vi "rsidr_core_global.vi"() -> ()   [LabVIEW 2020, in "Rohde&Schwarz CMWXP NR FR1 Measurement.lvlib"] (continued)
position\n\n<10_MErrPeakHighLimCheck>\n limit check result\nMagnitude error peak value, high EVM window position\n\n<11_PErr_RMSlowLimCheck>\n limit check result\nPhase error RMS value, low EVM window position\n\n<12_PErr_RMShLimCheck>\n limit check result\nPhase error RMS value, high EVM window position\n\n<13_PErrPeakLowLimCheck>\n limit check result\nPhase error peak value, low EVM window position\n\n<14_PErrPeakHighLimCheck>\n limit check result\nPhase error peak value, high EVM window position\n\n<15_IQoffsetLimCheck>\n limit check result\nI/Q origin offset\n\n<16_FreqErrorLimCheck>\n limit check result\nCarrier frequency error\n\n<17_TimingErrorLimCheck>\n limit check result\nTransmit time error\n\n<18_TXpowerLimCheck>\n limit check result\nUser equipment power\n\n<19_PeakPowerLimCheck>\n limit check result\nUser equipment peak power\n\n<20_RBpowerLimCheck>\n limit check result\nRB power\n\n<21_EVM_DMRSlLimCheck>\n limit check result\nEVM DMRS value, low EVM window position\n\n<22_EVM_DMRShLimCheck>\n limit check result\nEVM DMRS value, high EVM window position\n\n<23_MErr_DMRSlLimCheck>\n limit check result\nMagnitude error DMRS value, low EVM window position\n\n<24_MErr_DMRShLimCheck>\n limit check result\nMagnitude error DMRS value, high EVM window position\n\n<25_PErr_DMRSLimCheck>\n limit check result\nPhase error DMRS value, low EVM window position\n\n<26_PErr_DMRShLimCheck>\n limit check result\nPhase error DMRS value, high EVM window position\n\n<27_FreqErrorPpmLimCheck>\n limit check result\nCarrier frequency error in ppm\n\n<28_SampleClockELimCheck>\n limit check result\nSample clock error\n\nAvailable Repeated Capabilities:\ninstance: i0, i1, i2, i3, i4, i5, i6, i7, i8, i9, i10, i11, i12, i13, i14, i15, i16, i17, i18, i19, i20, i21, i22, i23, i24, i25, i26, i27, i28, i29, i30, i31, i32\r\n\nRemote-control command(s):\nCALCulate:NRSub:MEAS<i>:MEValuation:MODulation:CURRent?"}, {"Level"=4, "Class Only"=FALSE, "Identifier"="RSCMWXPNRFR1M_ATTR_QUERY_MULTI_EVAL_MEAS_MODULATION_AVERAGE_LIMIT_CHECK_RESULTS", "Descriptive Name"="Query Multi Eval Meas Modulation Average Limit Check Results", "Data Type"=enum."RawString", "Command"="CALC:NRS:MEAS{instance}:MEV:MOD:AVER?", "Access"=enum."Read Only", "Range Table"="", "Read Callback"="", "Write Callback"="", "Range Callback"="", "Check Callback"="", "Rngtable Callback"="", "Coerce Callback"="", "Supported Models"="", "Instrument Options"="", "Check Status Callback"="", "Flags"=0, "Help"="Return the average single value limit check results.\n\nReturn values:  \n<1_Reliability>\n decimal\n\n<2_OutOfTol>\n decimal\nOut of tolerance result, i.e. percentage of measurement intervals of the statistic count for modulation measurements exceeding the specified modulation limits.\n\n<3_EVM_RMSlowLimCheck>\n limit check result\nEVM RMS value, low EVM window position\n\n<4_EVM_RMShighLimCheck>\n limit check result\nEVM RMS value, high EVM window position\n\n<5_EVMpeakLowLimCheck>\n limit check result\nEVM peak value, low EVM window position\n\n<6_EVMpeakHighLimCheck>\n limit check result\nEVM peak value, high EVM window position\n\n<7_MErr_RMSlowLimCheck>\n limit check result\nMagnitude error RMS value, low EVM window position\n\n<8_MErr_RMShighLimCheck>\n limit check result\nMagnitude error RMS value, high EVM window position\n\n<9_MErrPeakLowLimCheck>\n limit check result\nMagnitude error peak value, low EVM window position\n\n<10_MErrPeakHighLimCheck>\n limit check result\nMagnitude error peak value, high EVM window position\n\n<11_PErr_RMSlowLimCheck>\n limit check result\nPhase error RMS value, low EVM window position\n\n<12_PErr_RMShLimCheck>\n limit check result\nPhase error RMS value, high EVM window position\n\n<13_PErrPeakLowLimCheck>\n limit check result\nPhase error peak value, low EVM window position\n\n<14_PErrPeakHighLimCheck>\n limit check result\nPhase error peak value, high EVM window position\n\n<15_IQoffsetLimCheck>\n limit check result\nI/Q origin offset\n\n<16_FreqErrorLimCheck>\n limit check result\nCarrier frequency error\n\n<17_TimingErrorLimCheck>\n limit check result\nTransmit time error\n\n<18_TXpowerLimCheck>\n limit check result\nUser equipment power\n\n<19_PeakPowerLimCheck>\n limit check result\nUser equipment peak power\n\n<20_RBpowerLimCheck>\n limit check result\nRB power\n\n<21_EVM_DMRSlLimCheck>\n limit check result\nEVM DMRS value, low EVM window position\n\n<22_EVM_DMRShLimCheck>\n limit check result\nEVM DMRS value, high EVM window position\n\n<23_MErr_DMRSlLimCheck>\n limit check result\nMagnitude error DMRS value, low EVM window position\n\n<24_MErr_DMRShLimCheck>\n limit check result\nMagnitude error DMRS value, high EVM window position\n\n<25_PErr_DMRSLimCheck>\n limit check result\nPhase error DMRS value, low EVM window position\n\n<26_PErr_DMRShLimCheck>\n limit check result\nPhase error DMRS value, high EVM window position\n\n<27_FreqErrorPpmLimCheck>\n limit check result\nCarrier frequency error in ppm\n\n<28_SampleClockELimCheck>\n limit check result\nSample clock error\n\nAvailable Repeated Capabilities:\ninstance: i0, i1, i2, i3, i4, i5, i6, i7, i8, i9, i10, i11, i12, i13, i14, i15, i16, i17, i18, i19, i20, i21, i22, i23, i24, i25, i26, i27, i28, i29, i30, i31, i32\r\n\nRemote-control command(s):\nCALCulate:NRSub:MEAS<i>:MEValuation:MODulation:AVERage?"}, {"Level"=4, "Class Only"=FALSE, "Identifier"="RSCMWXPNRFR1M_ATTR_READ_MULTI_EVAL_MEAS_MODULATION_EXTREME_RESULTS", "Descriptive Name"="Read Multi Eval Meas Modulation Extreme Results", "Data Type"=enum."RawString", "Command"="READ:NRS:MEAS{instance}:MEV:MOD:EXTR?", "Access"=enum."Read Only", "Range Table"="", "Read Callback"="", "Write Callback"="", "Range Callback"="", "Check Callback"="", "Rngtable Callback"="", "Coerce Callback"="", "Supported Models"="", "Instrument Options"="", "Check Status Callback"="", "Flags"=0, "Help"="Return the extreme single value results.\n\nReturn values:  \n<1_Reliability>\n decimal\n\n<2_OutOfTol>\n decimal\nOut of tolerance result, i.e. percentage of measurement intervals of the statistic count for modulation measurements exceeding the specified modulation limits.\nDefault unit:  % \n\n<3_EVM_RMSlow>\n float\nEVM RMS value, low EVM window position\nDefault unit:  % \n\n<4_EVM_RMShigh>\n float\nEVM RMS value, high EVM window position\nDefault unit:  % \n\n<5_EVMpeakLow>\n float\nEVM peak value, low EVM window position\nDefault unit:  %\n\n<6_EVMpeakHigh>\n float\nEVM peak value, high EVM window position\nDefault unit:  %\n\n<7_MErr_RMSlow>\n float\nMagnitude error RMS value, low EVM window position\nDefault unit:  %\n\n<8_MErr_RMShigh>\n float\nMagnitude error RMS value, high EVM window position\nDefault unit:  %\n\n<9_MErrPeakLow>\n float\nMagnitude error peak value, low EVM window position\nDefault unit:  %\n\n<10_MErrPeakHigh>\n float\nMagnitude error peak value, high EVM window position\nDefault unit:  %\n\n<11_PErr_RMSlow>\n float\nPhase error RMS value, low EVM window position\nDefault unit:  deg\n\n<12_PErr_RMSh>\n float\nPhase error RMS value, high EVM window position\nDefault unit:  deg\n\n<13_PErrPeakLow>\n float\nPhase error peak value, low EVM window position\nDefault unit:  deg\n\n<14_PErrPeakHigh>\n float\nPhase error peak value, high EVM window position\nDefault unit:  deg\n\n<15_IQoffset>\n float\nI/Q origin offset\nDefault unit:  dBc\n\n<16_FreqError>\n float\nCarrier frequency error\nDefault unit:  Hz\n\n<17_TimingError>\n float\nTransmit time error\nDefault unit:  Ts (basic time unit)\n\n<18_TXpowerMin>\n float\nMinimum user equipment power\nDefault unit:  dBm\n\n<19_TXpowerMax>\n float\nMaximum user equipment power\nDefault unit:  dBm\n\n<20_PeakPowerMin>\n float\nMinimum user equipment peak power\nDefault unit:  dBm\n\n<21_PeakPowerMax>\n float\nMaximum user equipment peak power\nDefault unit:  dBm\n\n<22_RBpowerMin>\n float\nMinimum RB power\nDefault unit:  dBm\n\n<23_RBpowerMax>\n float\nMaximum RB power\nDefault unit:  dBm\n\n<24_EVM_DMRSl>\n float\nEVM DMRS value, low EVM window position\nDefault unit:  %\n\n<25_EVM_DMRSh>\n float\nEVM DMRS value, high EVM window position\nDefault unit:  %\n\n<26_MErr_DMRSl>\n float\nMagnitude error DMRS value, low EVM window position\nDefault unit:  %\n\n<27_MErr_DMRSh>\n float\nMagnitude error DMRS value, high EVM window position\nDefault unit:  %\n\n<28_PErr_DMRS>\n float\nPhase error DMRS value, low EVM window position\nDefault unit:  deg\n\n<29_PErr_DMRSh>\n float\nPhase error DMRS value, high EVM window position\nDefault unit:  deg\n\n<30_FreqErrorPpm>\n float\nCarrier frequency error in ppm\nDefault unit:  ppm\n\n<31_SampleClockE>\n float\nSample clock error\nDefault unit:  ppm\n\nAvailable Repeated Capabilities:\ninstance: i0, i1, i2, i3, i4, i5, i6, i7, i8, i9, i10, i11, i12, i13, i14, i15, i16, i17, i18, i19, i20, i21, i22, i23, i24, i25, i26, i27, i28, i29, i30, i31, i32\r\n\nRemote-control command(s):\nREAD:NRSub:MEAS<i>:MEValuation:MODulation:EXTReme?"}, {"Level"=4, "Class Only"=FALSE, "Identifier"="RSCMWXPNRFR1M_ATTR_FETCH_MULTI_EVAL_MEAS_MODULATION_EXTREME_RESULTS", "Descriptive Name"="Fetch Multi Eval Meas Modulation Extreme Results", "Data Type"=enum."RawString", "Command"="FETC:NRS:MEAS{instance}:MEV:MOD:EXTR?", "Access"=enum."Read Only", "Range Table"="", "Read Callback"="", "Write Callback"="", "Range Callback"="", "Check Callback"="", "Rngtable Callback"="", "Coerce Callback"="", "Supported Models"="", "Instrument Options"="", "Check Status Callback"="", "Flags"=0, "Help"="Return the extreme single value results.\n\nReturn values:  \n<1_Reliability>\n decimal\n\n<2_OutOfTol>\n decimal\nOut of tolerance result, i.e. percentage of measurement intervals of the statistic count for modulation measurements exceeding the specified modulation limits.\nDefault unit:  % \n\n<3_EVM_RMSlow>\n float\nEVM RMS value, low EVM window position\nDefault unit:  % \n\n<4_EVM_RMShigh>\n float\nEVM RMS value, high EVM window position\nDefault unit:  % \n\n<5_EVMpeakLow>\n float\nEVM peak value, low EVM window position\nDefault unit:  %\n\n<6_EVMpeakHigh>\n float\nEVM peak value, high EVM window position\nDefault unit:  %\n\n<7_MErr_RMSlow>\n float\nMagnitude error RMS value, low EVM window position\nDefault unit:  %\n\n<8_MErr_RMShigh>\n float\nMagnitude error RMS value, high EVM window position\nDefault unit:  %\n\n<9_MErrPeakLow>\n float\nMagnitude error peak value, low EVM window position\nDefault unit:  %\n\n<10_MErrPeakHigh>\n float\nMagnitude error peak value, high EVM window position\nDefault unit:  %\n\n<11_PErr_RMSlow>\n float\nPhase error RMS value, low EVM window position\nDefault unit:  deg\n\n<12_PErr_RMSh>\n float\nPhase error RMS value, high EVM window position\nDefault unit:  deg\n\n<13_PErrPeakLow>\n float\nPhase error peak value, low EVM window position\nDefault unit:  deg\n\n<14_PErrPeakHigh>\n float\nPhase error peak value, high EVM window position\nDefault unit:  deg\n\n<15_IQoffset>\n float\nI/Q origin offset\nDefault unit:  dBc\n\n<16_FreqError>\n float\nCarrier frequency error\nDefault unit:  Hz\n\n<17_TimingError>\n float\nTransmit time error\nDefault unit:  Ts (basic time unit)\n\n<18_TXpowerMin>\n float\nMinimum user equipment power\nDefault unit:  dBm\n\n<19_TXpowerMax>\n float\nMaximum user equipment power\nDefault unit:  dBm\n\n<20_PeakPowerMin>\n float\nMinimum user equipment peak power\nDefault unit:  dBm\n\n<21_PeakPowerMax>\n float\nMaximum user equipment peak power\nDefault unit:  dBm\n\n<22_RBpowerMin>\n float\nMinimum RB power\nDefault unit:  dBm\n\n<23_RBpowerMax>\n float\nMaximum RB power\nDefault unit:  dBm\n\n<24_EVM_DMRSl>\n float\nEVM DMRS value, low EVM window position\nDefault unit:  %\n\n<25_EVM_DMRSh>\n float\nEVM DMRS value, high EVM window position\nDefault unit:  %\n\n<26_MErr_DMRSl>\n float\nMagnitude error DMRS value, low EVM window position\nDefault unit:  %\n\n<27_MErr_DMRSh>\n float\nMagnitude error DMRS value, high EVM window position\nDefault unit:  %\n\n<28_PErr_DMRS>\n float\nPhase error DMRS value, low EVM window position\nDefault unit:  deg\n\n<29_PErr_DMRSh>\n float\nPhase error DMRS value, high EVM window position\nDefault unit:  deg\n\n<30_FreqErrorPpm>\n float\nCarrier frequency error in ppm\nDefault unit:  ppm\n\n<31_SampleClockE>\n float\nSample clock error\nDefault unit:  ppm\n\nAvailable Repeated Capabilities:\ninstance: i0, i1, i2, i3, i4, i5, i6, i7, i8, i9, i10, i11, i12, i13, i14, i15, i16, i17, i18, i19, i20, i21, i22, i23, i24, i25, i26, i27, i28, i29, i30, i31, i32\r\n\nRemote-control command(s):\nFETCh:NRSub:MEAS<i>:MEValuation:MODulation:EXTReme?"}, {"Level"=4, "Class Only"=FALSE, "Identifier"="RSCMWXPNRFR1M_ATTR_QUERY_MULTI_EVAL_MEAS_MODULATION_EXTREME_LIMIT_CHECK_RESULTS", "Descriptive Name"="Query Multi Eval Meas Modulation Extreme Limit Check Results", "Data Type"=enum."RawString", "Command"="CALC:NRS:MEAS{instance}:MEV:MOD:EXTR?", "Access"=enum."Read Only", "Range Table"="", "Read Callback"="", "Write Callback"="", "Range Callback"="", "Check Callback"="", "Rngtable Callback"="", "Coerce Callback"="", "Supported Models"="", "Instrument Options"="", "Check Status Callback"="", "Flags"=0, "Help"="Return the extreme single value limit check results.\n\nReturn values:  \n<1_Reliability>\n decimal\n\n<2_OutOfTol>\n decimal\nOut of tolerance result, i.e. percentage of measurement intervals of the statistic count for modulation measurements exceeding the specified modulation limits.\nDefault unit:  % \n\n<3_EVM_RMSlowLimCheck>\n limit check result\nEVM RMS value, low EVM window position\n\n<4_EVM_RMShighLimCheck>\n limit check result\nEVM RMS value, high EVM window position\n\n<5_EVMpeakLowLimCheck>\n limit check result\nEVM peak value, low EVM window position\n\n<6_EVMpeakHighLimCheck>\n limit check result\nEVM peak value, high EVM window position\n\n<7_MErr_RMSlowLimCheck>\n limit check result\nMagnitude error RMS value, low EVM window position\n\n<8_MErr_RMShighLimCheck>\n limit check result\nMagnitude error RMS value, high EVM window position\n\n<9_MErrPeakLowLimCheck>\n limit check result\nMagnitude error peak value, low EVM window position\n\n<10_MErrPeakHighLimCheck>\n limit check result\nMagnitude error peak value, high EVM window position\n\n<11_PErr_RMSlowLimCheck>\n limit check result\nPhase error RMS value, low EVM window position\n\n<12_PErr_RMShLimCheck>\n limit check result\nPhase error RMS value, high EVM window position\n\n<13_PErrPeakLowLimCheck>\n limit check result\nPhase error peak value, low EVM window position\n\n<14_PErrPeakHighLimCheck>\n limit check result\nPhase error peak value, high EVM window position\n\n<15_IQoffsetLimCheck>\n limit check result\nI/Q origin offset\n\n<16_FreqErrorLimCheck>\n limit check result\nCarrier frequency error\n\n<17_TimingErrorLimCheck>\n limit check result\nTransmit time error\n\n<18_TXpowerMinLimCheck>\n limit check result\nMinimum user equipment power\n\n<19_TXpowerMaxLimCheck>\n limit check result\nMaximum user equipment power\n\n<20_PeakPowerMinLimCheck>\n limit check result\nMinimum user equipment peak power\n\n<21_PeakPowerMaxLimCheck>\n limit check result\nMaximum user equipment peak power\n\n<22_RBpowerMinLimCheck>\n limit check result\nMinimum RB power\n\n<23_RBpowerMaxLimCheck>\n limit check result\nMaximum RB power\n\n<24_EVM_DMRSlLimCheck>\n limit check result\nEVM DMRS value, low EVM window position\n\n<25_EVM_DMRShLimCheck>\n limit check result\nEVM DMRS value, high EVM window position\n\n<26_MErr_DMRSlLimCheck>\n limit check result\nMagnitude error DMRS value, low EVM window position\n\n<27_MErr_DMRShLimCheck>\n limit check result\nMagnitude error DMRS value, high EVM window position\n\n<28_PErr_DMRSLimCheck>\n limit check result\nPhase error DMRS value, low EVM window position\n\n<29_PErr_DMRShLimCheck>\n limit check result\nPhase error DMRS value, high EVM window position\n\n<30_FreqErrorPpmLimCheck>\n limit check result\nCarrier frequency error in ppm\n\n<31_SampleClockELimCheck>\n limit check result\nSample clock error\n\nAvailable Repeated Capabilities:\ninstance: i0, i1, i2, i3, i4, i5, i6, i7, i8, i9, i10, i11, i12, i13, i14, i15, i16, i17, i18, i19, i20, i21, i22, i23, i24, i25, i26, i27, i28, i29, i30, i31, i32\r\n\nRemote-control command(s):\nCALCulate:NRSub:MEAS<i>:MEValuation:MODulation:EXTReme?"}, {"Level"=3, "Class Only"=TRUE, "Identifier"="", "Descriptive Name"="Power Monitor", "Data Type"=enum."ViInt32", "Command"="", "Access"=enum."Read Only", "Range Table"="", "Read Callback"="", "Write Callback"="", "Range Callback"="", "Check Callback"="", "Rngtable Callback"="", "Coerce Callback"="", "Supported Models"="", "Instrument Options"="", "Check Status Callback"="", "Flags"=0, "Help"="The commands in this class return the power monitor results."}, {"Level"=4, "Class Only"=FALSE, "Identifier"="RSCMWXPNRFR1M_ATTR_READ_MULTI_EVAL_MEAS_TRACE_POWER_MONITOR_RESULTS", "Descriptive Name"="Read Multi Eval Meas Trace Power Monitor Results", "Data Type"=enum."RawString", "Command"="READ:NRS:MEAS{instance}:MEV:TRAC:PMON?", "Access"=enum."Read Only", "Range Table"="", "Read Callback"="", "Write Callback"="", "Range Callback"="", "Check Callback"="", "Rngtable Callback"="", "Coerce Callback"="", "Supported Models"="", "Instrument Options"="", "Check Status Callback"="", "Flags"=0, "Help"="Returns the power monitor results for all captured subframes.\n\nReturn values:  \n<Reliability>\n decimal\n\n<Power>\n float\nComma-separated list of power values, one value per subframe\nDefault unit:  dBm\n\nAvailable Repeated Capabilities:\ninstance: i0, i1, i2, i3, i4, i5, i6, i7, i8, i9, i10, i11, i12, i13, i14, i15, i16, i17, i18, i19, i20, i21, i22, i23, i24, i25, i26, i27, i28, i29, i30, i31, i32\r\n\nRemote-control command(s):\nREAD:NRSub:MEAS<i>:MEValuation:TRACe:PMONitor?"}, {"Level"=4, "Class Only"=FALSE, "Identifier"="RSCMWXPNRFR1M_ATTR_FETCH_MULTI_EVAL_MEAS_TRACE_POWER_MONITOR_RESULTS", "Descriptive Name"="Fetch Multi Eval Meas Trace Power Monitor Results", "Data Type"=enum."RawString", "Command"="FETC:NRS:MEAS{instance}:MEV:TRAC:PMON?", "Access"=enum."Read Only", "Range Table"="", "Read Callback"="", "Write Callback"="", "Range Callback"="", "Check Callback"="", "Rngtable Callback"="", "Coerce Callback"="", "Supported Models"="", "Instrument Options"="", "Check Status Callback"="", "Flags"=0, "Help"="Returns the power monitor results for all captured subframes.\n\nReturn values:  \n<Reliability>\n decimal\n\n<Power>\n float\nComma-separated list of power values, one value per subframe\nDefault unit:  dBm\n\nAvailable Repeated Capabilities:\ninstance: i0, i1, i2, i3, i4, i5, i6, i7, i8, i9, i10, i11, i12, i13, i14, i15, i16, i17, i18, i19, i20, i21, i22, i23, i24, i25, i26, i27, i28, i29, i30, i31, i32\r\n\nRemote-control command(s):\nFETCh:NRSub:MEAS<i>:MEValuation:TRACe:PMONitor?"}, {"Level"=4, "Class Only"=FALSE, "Identifier"="RSCMWXPNRFR1M_ATTR_READ_MULTI_EVAL_MEAS_POWER_MONITOR_CURRENT_RESULTS", "Descriptive Name"="Read Multi Eval Meas Power Monitor Current Results", "Data Type"=enum."RawString", "Command"="READ:NRS:MEAS{instance}:MEV:PMON:CURR?", "Access"=enum."Read Only", "Range Table"="", "Read Callback"="", "Write Callback"="", "Range Callback"="", "Check Callback"="", "Rngtable Callback"="", "Coerce Callback"="", "Supported Models"="", "Instrument Options"="", "Check Status Callback"="", "Flags"=0, "Help"="Returns the current total TX power.\n\nReturn values:  \n<Reliability>\n decimal\n\n<OutOfTolerance>\n decimal\nOut of tolerance result, i.e. percentage of measurement intervals of the statistic count for power measurements exceeding the specified power limits.\nDefault unit:  % \n\n<TXpower>\n float\nTotal TX power\nDefault unit:  dBm\n\nAvailable Repeated Capabilities:\ninstance: i0, i1, i2, i3, i4, i5, i6, i7, i8, i9, i10, i11, i12, i13, i14, i15, i16, i17, i18, i19, i20, i21, i22, i23, i24, i25, i26, i27, i28, i29, i30, i31, i32\r\n\nRemote-control command(s):\nREAD:NRSub:MEAS<i>:MEValuation:PMONitor:CURRent?"}, {"Level"=4, "Class Only"=FALSE, "Identifier"="RSCMWXPNRFR1M_ATTR_READ_MULTI_EVAL_MEAS_POWER_MONITOR_AVERAGE_RESULTS", "Descriptive Name"="Read Multi Eval Meas Power Monitor Average Results", "Data Type"=enum."RawString", "Command"="READ:NRS:MEAS{instance}:MEV:PMON:AVER?", "Access"=enum."Read Only", "Range Table"="", "Read Callback"="", "Write Callback"="", "Range Callback"="", "Check Callback"="", "Rngtable Callback"="", "Coerce Callback"="", "Supported Models"="", "Instrument Options"="", "Check Status Callback"="", "Flags"=0, "Help"="Returns the average total TX power.\n\nReturn values:  \n<Reliability>\n decimal\n\n<OutOfTolerance>\n decimal\nOut of tolerance result, i.e. percentage of measurement intervals of the statistic count for power measurements exceeding the specified power limits.\nDefault unit:  % \n\n<TXpower>\n float\nTotal TX power\nDefault unit:  dBm\n\nAvailable Repeated Capabilities:\ninstance: i0, i1, i2, i3, i4, i5, i6, i7, i8, i9, i10, i11, i12, i13, i14, i15, i16, i17, i18, i19, i20, i21, i22, i23, i24, i25, i26, i27, i28, i29, i30, i31, i32\r\n\nRemote-control command(s):\nREAD:NRSub:MEAS<i>:MEValuation:PMONitor:AVERage?"}, {"Level"=4, "Class Only"=FALSE, "Identifier"="RSCMWXPNRFR1M_ATTR_READ_MULTI_EVAL_MEAS_POWER_MONITOR_STANDARD_DEVIATION_RESULTS", "Descriptive Name"="Read Multi Eval Meas Power Monitor Standard Deviation Results", "Data Type"=enum."RawString", "Command"="READ:NRS:MEAS{instance}:MEV:PMON:SDEV?", "Access"=enum."Read Only", "Range Table"="", "Read Callback"="", "Write Callback"="", "Range Callback"="", "Check Callback"="", "Rngtable Callback"="", "Coerce Callback"="", "Supported Models"="", "Instrument Options"="", "Check Status Callback"="", "Flags"=0, "Help"="Returns the standard deviation total TX power.\n\nReturn values:  \n<Reliability>\n decimal\n\n<OutOfTolerance>\n decimal\nOut of tolerance result, i.e. percentage of measurement intervals of the statistic count for power measurements exceeding the specified power limits.\nDefault unit:  % \n\n<TXpower>\n float\nTotal TX power\nDefault unit:  dBm\n\nAvailable Repeated Capabilities:\ninstance: i0, i1, i2, i3, i4, i5, i6, i7, i8, i9, i10, i11, i12, i13, i14, i15, i16, i17, i18, i19, i20, i21, i22, i23, i24, i25, i26, i27, i28, i29, i30, i31, i32\r\n\nRemote-control command(s):\nREAD:NRSub:MEAS<i>:MEValuation:PMONitor:SDEViation?"}, {"Level"=4, "Class Only"=FALSE, "Identifier"="RSCMWXPNRFR1M_ATTR_READ_MULTI_EVAL_MEAS_POWER_MONITOR_MAXIMUM_RESULTS", "Descriptive Name"="Read Multi Eval Meas Power Monitor Maximum Results", "Data Type"=enum."RawString", "Command"="READ:NRS:MEAS{instance}:MEV:PMON:MAX?", "Access"=enum."Read Only", "Range Table"="", "Read Callback"="", "Write Callback"="", "Range Callback"="", "Check Callback"="", "Rngtable Callback"="", "Coerce Callback"="", "Supported Models"="", "Instrument Options"="", "Check Status Callback"="", "Flags"=0, "Help"="Returns the maximum total TX power.\n\nReturn values:  \n<Reliability>\n decimal\n\n<OutOfTolerance>\n decimal\nOut of tolerance result, i.e. percentage of measurement intervals of the statistic count for power measurements exceeding the specified power limits.\nDefault unit:  % \n\n<TXpower>\n float\nTotal TX power\nDefault unit:  dBm\n\nAvailable Repeated Capabilities:\ninstance: i0, i1, i2, i3, i4, i5, i6, i7, i8, i9, i10, i11, i12, i13, i14, i15, i16, i17, i18, i19, i20, i21, i22, i23, i24, i25, i26, i27, i28, i29, i30, i31, i32\r\n\nRemote-control command(s):\nREAD:NRSub:MEAS<i>:MEValuation:PMONitor:MAXimum?"}, {"Level"=4, "Class Only"=FALSE, "Identifier"="RSCMWXPNRFR1M_ATTR_READ_MULTI_EVAL_MEAS_POWER_MONITOR_MINIMUM_RESULTS", "Descriptive Name"="Read Multi Eval Meas Power Monitor Minimum Results", "Data Type"=enum."RawString", "Command"="READ:NRS:MEAS{instance}:MEV:PMON:MIN?", "Access"=enum."Read Only", "Range Table"="", "Read Callback"="", "Write Callback"="", "Range Callback"="", "Check Callback"="", "Rngtable Callback"="", "Coerce Callback"="", "Supported Models"="", "Instrument Options"="", "Check Status Callback"="", "Flags"=0, "Help"="Returns the minimum total TX power.\n\nReturn values:  \n<Reliability>\n decimal\n\n<OutOfTolerance>\n decimal\nOut of tolerance result, i.e. percentage of measurement intervals of the statistic count for power measurements exceeding the specified power limits.\nDefault unit:  % \n\n<TXpower>\n float\nTotal TX power\nDefault unit:  dBm\n\nAvailable Repeated Capabilities:\ninstance: i0, i1, i2, i3, i4, i5, i6, i7, i8, i9, i10, i11, i12, i13, i14, i15, i16, i17, i18, i19, i20, i21, i22, i23, i24, i25, i26, i27, i28, i29, i30, i31, i32\r\n\nRemote-control command(s):\nREAD:NRSub:MEAS<i>:MEValuation:PMONitor:MINimum?"}, {"Level"=4, "Class Only"=FALSE, "Identifier"="RSCMWXPNRFR1M_ATTR_FETCH_MULTI_EVAL_MEAS_POWER_MONITOR_CURRENT_RESULTS", "Descriptive Name"="Fetch Multi Eval Meas Power Monitor Current Results", "Data Type"=enum."RawString", "Command"="FETC:NRS:MEAS{instance}:MEV:PMON:CURR?", "Access"=enum."Read Only", "Range Table"="", "Read Callback"="", "Write Callback"="", "Range Callback"="", "Check Callback"="", "Rngtable Callback"="", "Coerce Callback"="", "Supported Models"="", "Instrument Options"="", "Check Status Callback"="", "Flags"=0, "Help"="Returns the current total TX power.\n\nReturn values:  \n<Reliability>\n decimal\n\n<OutOfTolerance>\n decimal\nOut of tolerance result, i.e. percentage of measurement intervals of the statistic count for power measurements exceeding the specified power limits.\nDefault unit:  % \n\n<TXpower>\n float\nTotal TX power\nDefault unit:  dBm\n\nAvailable Repeated Capabilities:\ninstance: i0, i1, i2, i3, i4, i5, i6, i7, i8, i9, i10, i11, i12, i13, i14, i15, i16, i17, i18, i19, i20, i21, i22, i23, i24, i25, i26, i27, i28, i29, i30, i31, i32\r\n\nRemote-control command(s):\nFETCh:NRSub:MEAS<i>:MEValuation:PMONitor:CURRent?"}, {"Level"=4, "Class Only"=FALSE, "Identifier"="RSCMWXPNRFR1M_ATTR_FETCH_MULTI_EVAL_MEAS_POWER_MONITOR_AVERAGE_RESULTS", "Descriptive Name"="Fetch Multi Eval Meas Power Monitor Average Results", "Data Type"=enum."RawString", "Command"="FETC:NRS:MEAS{instance}:MEV:PMON:AVER?", "Access"=enum."Read Only", "Range Table"="", "Read Callback"="", "Write Callback"="", "Range Callback"="", "Check Callback"="", "Rngtable Callback"="", "Coerce Callback"="", "Supported Models"="", "Instrument Options"="", "Check Status Callback"="", "Flags"=0, "Help"="Returns the average total TX power.\n\nReturn values:  \n<Reliability>\n decimal\n\n<OutOfTolerance>\n decimal\nOut of tolerance result, i.e. percentage of measurement intervals of the statistic count for power measurements exceeding the specified power limits.\nDefault unit:  % \n\n<TXpower>\n float\nTotal TX power\nDefault unit:  dBm\n\nAvailable Repeated Capabilities:\ninstance: i0, i1, i2, i3, i4, i5, i6, i7, i8, i9, i10, i11, i12, i13, i14, i15, i16, i17, i18, i19, i20, i21, i22, i23, i24, i25, i26, i27, i28, i29, i30, i31, i32\r\n\nRemote-control command(s):\nFETCh:NRSub:MEAS<i>:MEValuation:PMONitor:AVERage?"}, {"Level"=4, "Class Only"=FALSE, "Identifier"="RSCMWXPNRFR1M_ATTR_FETCH_MULTI_EVAL_MEAS_POWER_MONITOR_STANDARD_DEVIATION_RESULTS", "Descriptive Name"="Fetch Multi Eval Meas Power Monitor Standard Deviation Results", "Data Type"=enum."RawString", "Command"="FETC:NRS:MEAS{instance}:MEV:PMON:SDEV?", "Access"=enum."Read Only", "Range Table"="", "Read Callback"="", "Write Callback"="", "Range Callback"="", "Check Callback"="", "Rngtable Callback"="", "Coerce Callback"="", "Supported Models"="", "Instrument Options"="", "Check Status Callback"="", "Flags"=0, "Help"="Returns the standard deviation total TX power.\n\nReturn values:  \n<Reliability>\n decimal\n\n<OutOfTolerance>\n decimal\nOut of tolerance result, i.e. percentage of measurement intervals of the statistic count for power measurements exceeding the specified power limits.\nDefault unit:  % \n\n<TXpower>\n float\nTotal TX power\nDefault unit:  dBm\n\nAvailable Repeated Capabilities:\ninstance: i0, i1, i2, i3, i4, i5, i6, i7, i8, i9, i10, i11, i12, i13, i14, i15, i16, i17, i18, i19, i20, i21, i22, i23, i24, i25, i26, i27, i28, i29, i30, i31, i32\r\n\nRemote-control command(s):\nFETCh:NRSub:MEAS<i>:MEValuation:PMONitor:SDEViation?"}, {"Level"=4, "Class Only"=FALSE, "Identifier"="RSCMWXPNRFR1M_ATTR_FETCH_MULTI_EVAL_MEAS_POWER_MONITOR_MAXIMUM_RESULTS", "Descriptive Name"="Fetch Multi Eval Meas Power Monitor Maximum Results", "Data Type"=enum."RawString", "Command"="FETC:NRS:MEAS{instance}:MEV:PMON:MAX?", "Access"=enum."Read Only", "Range Table"="", "Read Callback"="", "Write Callback"="", "Range Callback"="", "Check Callback"="", "Rngtable Callback"="", "Coerce Callback"="", "Supported Models"="", "Instrument Options"="", "Check Status Callback"="", "Flags"=0, "Help"="Returns the maximum total TX power.\n\nReturn values:  \n<Reliability>\n decimal\n\n<OutOfTolerance>\n decimal\nOut of tolerance result, i.e. percentage of measurement intervals of the statistic count for power measurements exceeding the specified power limits.\nDefault unit:  % \n\n<TXpower>\n float\nTotal TX power\nDefault unit:  dBm\n\nAvailable Repeated Capabilities:\ninstance: i0, i1, i2, i3, i4, i5, i6, i7, i8, i9, i10, i11, i12, i13, i14, i15, i16, i17, i18, i19, i20, i21, i22, i23, i24, i25, i26, i27, i28, i29, i30, i31, i32\r\n\nRemote-control command(s):\nFETCh:NRSub:MEAS<i>:MEValuation:PMONitor:MAXimum?"}, {"Level"=4, "Class Only"=FALSE, "Identifier"="RSCMWXPNRFR1M_ATTR_FETCH_MULTI_EVAL_MEAS_POWER_MONITOR_MINIMUM_RESULTS", "Descriptive Name"="Fetch Multi Eval Meas Power Monitor Minimum Results", "Data Type"=enum."RawString", "Command"="FETC:NRS:MEAS{instance}:MEV:PMON:MIN?", "Access"=enum."Read Only", "Range Table"="", "Read Callback"="", "Write Callback"="", "Range Callback"="", "Check Callback"="", "Rngtable Callback"="", "Coerce Callback"="", "Supported Models"="", "Instrument Options"="", "Check Status Callback"="", "Flags"=0, "Help"="Returns the minimum total TX power.\n\nReturn values:  \n<Reliability>\n decimal\n\n<OutOfTolerance>\n decimal\nOut of tolerance result, i.e. percentage of measurement intervals of the statistic count for power measurements exceeding the specified power limits.\nDefault unit:  % \n\n<TXpower>\n float\nTotal TX power\nDefault unit:  dBm\n\nAvailable Repeated Capabilities:\ninstance: i0, i1, i2, i3, i4, i5, i6, i7, i8, i9, i10, i11, i12, i13, i14, i15, i16, i17, i18, i19, i20, i21, i22, i23, i24, i25, i26, i27, i28, i29, i30, i31, i32\r\n\nRemote-control command(s):\nFETCh:NRSub:MEAS<i>:MEValuation:PMONitor:MINimum?"}, {"Level"=3, "Class Only"=TRUE, "Identifier"="", "Descriptive Name"="Power Dynamics", "Data Type"=enum."ViInt32", "Command"="", "Access"=enum."Read Only", "Range Table"="", "Read Callback"="", "Write Callback"="", "Range Callback"="", "Check Callback"="", "Rngtable Callback"="", "Coerce Callback"="", "Supported Models"="", "Instrument Options"="", "Check Status Callback"="", "Flags"=0, "Help"="The commands in this class return the power dynamics measurement results."}, {"Level"=4, "Class Only"=FALSE, "Identifier"="RSCMWXPNRFR1M_ATTR_READ_MULTI_EVAL_MEAS_TRACE_POWER_DYNAMICS_CURRENT_RESULTS", "Descriptive Name"="Read Multi Eval Meas Trace Power Dynamics Current Results", "Data Type"=enum."RawString", "Command"="READ:NRS:MEAS{instance}:MEV:TRAC:PDYN:CURR?", "Access"=enum."Read Only", "Range Table"="", "Read Callback"="", "Write Callback"="", "Range Callback"="", "Check Callback"="", "Rngtable Callback"="", "Coerce Callback"="", "Supported Models"="", "Instrument Options"="", "Check Status Callback"="", "Flags"=0, "Help"="Return the values of the power dynamics traces. Each value is sampled with 48 Ts, corresponding to 1.5625 s. The results of the current trace is retrieved.\n\nReturn values:  \n<Reliability>\n decimal\n\n<Power>\n float\n2048 power values, from -1100 s to +2098.4375 s relative to the start of the measure subframe. The values have a spacing of 1.5625 s. The 705th value is at the start of the 'Measure Subframe' (0 s).\nThe diagram in the GUI shows only a subsection of this trace.\nDefault unit:  dBm\n\nAvailable Repeated Capabilities:\ninstance: i0, i1, i2, i3, i4, i5, i6, i7, i8, i9, i10, i11, i12, i13, i14, i15, i16, i17, i18, i19, i20, i21, i22, i23, i24, i25, i26, i27, i28, i29, i30, i31, i32\r\n\nRemote-control command(s):\nREAD:NRSub:MEAS<i>:MEValuation:TRACe:PDYNamics:CURRent?"}, {"Level"=4, "Class Only"=FALSE, "Identifier"="RSCMWXPNRFR1M_ATTR_READ_MULTI_EVAL_MEAS_TRACE_POWER_DYNAMICS_AVERAGE_RESULTS", "Descriptive Name"="Read Multi Eval Meas Trace Power Dynamics Average Results", "Data Type"=enum."RawString", "Command"="READ:NRS:MEAS{instance}:MEV:TRAC:PDYN:AVER?", "Access"=enum."Read Only", "Range Table"="", "Read Callback"="", "Write Callback"="", "Range Callback"="", "Check Callback"="", "Rngtable Callback"="", "Coerce Callback"="", "Supported Models"="", "Instrument Options"="", "Check Status Callback"="", "Flags"=0, "Help"="Return the values of the power dynamics traces. Each value is sampled with 48 Ts, corresponding to 1.5625 s. The results of the average trace is retrieved.\n\nReturn values:  \n<Reliability>\n decimal\n\n<Power>\n float\n2048 power values, from -1100 s to +2098.4375 s relative to the start of the measure subframe. The values have a spacing of 1.5625 s. The 705th value is at the start of the 'Measure Subframe' (0 s).\nThe diagram in the GUI shows only a subsection of this trace.\nDefault unit:  dBm\n\nAvailable Repeated Capabilities:\ninstance: i0, i1, i2, i3, i4, i5, i6, i7, i8, i9, i10, i11, i12, i13, i14, i15, i16, i17, i18, i19, i20, i21, i22, i23, i24, i25, i26, i27, i28, i29, i30, i31, i32\r\n\nRemote-control command(s):\nREAD:NRSub:MEAS<i>:MEValuation:TRACe:PDYNamics:AVERage?"}, {"Level"=4, "Class Only"=FALSE, "Identifier"="RSCMWXPNRFR1M_ATTR_READ_MULTI_EVAL_MEAS_TRACE_POWER_DYNAMICS_MAXIMUM_RESULTS", "Descriptive Name"="Read Multi Eval Meas Trace Power Dynamics Maximum Results", "Data Type"=enum."RawString", "Command"="READ:NRS:MEAS{instance}:MEV:TRAC:PDYN:MAX?", "Access"=enum."Read Only", "Range Table"="", "Read Callback"="", "Write Callback"="", "Range Callback"="", "Check Callback"="", "Rngtable Callback"="", "Coerce Callback"="", "Supported Models"="", "Instrument Options"="", "Check Status Callback"="", "Flags"=0, "Help"="Return the values of the power dynamics traces. Each value is sampled with 48 Ts, corresponding to 1.5625 s. The results of the maximum trace is retrieved.\n\nReturn values:  \n<Reliability>\n decimal\n\n<Power>\n float\n2048 power values, from -1100 s to +2098.4375 s relative to the start of the measure subframe. The values have a spacing of 1.5625 s. The 705th value is at the start of the 'Measure Subframe' (0 s).\nThe diagram in the GUI shows only a subsection of this trace.\nDefault unit:  dBm\n\nAvailable Repeated Capabilities:\ninstance: i0, i1, i2, i3, i4, i5, i6, i7, i8, i9, i10, i11, i12, i13, i14, i15, i16, i17, i18, i19, i20, i21, i22, i23, i24, i25, i26, i27, i28, i29, i30, i31, i32\r\n\nRemote-control command(s):\nREAD:NRSub:MEAS<i>:MEValuation:TRACe:PDYNamics:MAXimum?"}, {"Level"=4, "Class Only"=FALSE, "Identifier"="RSCMWXPNRFR1M_ATTR_FETCH_MULTI_EVAL_MEAS_TRACE_POWER_DYNAMICS_CURRENT_RESULTS", "Descriptive Name"="Fetch Multi Eval Meas Trace Power Dynamics Current Results", "Data Type"=enum."RawString", "Command"="FETC:NRS:MEAS{instance}:MEV:TRAC:PDYN:CURR?", "Access"=enum."Read Only", "Range Table"="", "Read Callback"="", "Write Callback"="", "Range Callback"="", "Check Callback"="", "Rngtable Callback"="", "Coerce Callback"="", "Supported Models"="", "Instrument Options"="", "Check Status Callback"="", "Flags"=0, "Help"="Return the values of the power dynamics traces. Each value is sampled with 48 Ts, corresponding to 1.5625 s. The results of the current trace is retrieved.\n\nReturn values:  \n<Reliability>\n decimal\n\n<Power>\n float\n2048 power values, from -1100 s to +2098.4375 s relative to the start of the measure subframe. The values have a spacing of 1.5625 s. The 705th value is at the start of the 'Measure Subframe' (0 s).\nThe diagram in the GUI shows only a subsection of this trace.\nDefault unit:  dBm\n\nAvailable Repeated Capabilities:\ninstance: i0, i1, i2, i3, i4, i5, i6, i7, i8, i9, i10, i11, i12, i13, i14, i15, i16, i17, i18, i19, i20, i21, i22, i23, i24, i25, i26, i27, i28, i29, i30, i31, i32\r\n\nRemote-control command(s):\nFETCh:NRSub:MEAS<i>:MEValuation:TRACe:PDYNamics:CURRent?"}, {"Level"=4, "Class Only"=FALSE, "Identifier"="RSCMWXPNRFR1M_ATTR_FETCH_MULTI_EVAL_MEAS_TRACE_POWER_DYNAMICS_AVERAGE_RESULTS", "Descriptive Name"="Fetch Multi Eval Meas Trace Power Dynamics Average Results", "Data Type"=enum."RawString", "Command"="FETC:NRS:MEAS{instance}:MEV:TRAC:PDYN:AVER?", "Access"=enum."Read Only", "Range Table"="", "Read Callback"="", "Write Callback"="", "Range Callback"="", "Check Callback"="", "Rngtable Callback"="", "Coerce Callback"="", "Supported Models"="", "Instrument Options"="", "Check Status Callback"="", "Flags"=0, "Help"="Return the values of the power dynamics traces. Each value is sampled with 48 Ts, corresponding to 1.5625 s. The results of the average trace is retrieved.\n\nReturn values:  \n<Reliability>\n decimal\n\n<Power>\n float\n2048 power values, from -1100 s to +2098.4375 s relative to the start of the measure subframe. The values have a spacing of 1.5625 s. The 705th value is at the start of the 'Measure Subframe' (0 s).\nThe diagram in the GUI shows only a subsection of this trace.\nDefault unit:  dBm\n\nAvailable Repeated Capabilities:\ninstance: i0, i1, i2, i3, i4, i5, i6, i7, i8, i9, i10, i11, i12, i13, i14, i15, i16, i17, i18, i19, i20, i21, i22, i23, i24, i25, i26, i27, i28, i29, i30, i31, i32\r\n\nRemote-control command(s):\nFETCh:NRSub:MEAS<i>:MEValuation:TRACe:PDYNamics:AVERage?"}, {"Level"=4, "Class Only"=FALSE, "Identifier"="RSCMWXPNRFR1M_ATTR_FETCH_MULTI_EVAL_MEAS_TRACE_POWER_DYNAMICS_MAXIMUM_RESULTS", "Descriptive Name"="Fetch Multi Eval Meas Trace Power Dynamics Maximum Results", "Data Type"=enum."RawString", "Command"="FETC:NRS:MEAS{instance}:MEV:TRAC:PDYN:MAX?", "Access"=enum."Read Only", "Range Table"="", "Read Callback"="", "Write Callback"="", "Range Callback"="", "Check Callback"="", "Rngtable Callback"="", "Coerce Callback"="", "Supported Models"="", "Instrument Options"="", "Check Status Callback"="", "Flags"=0, "Help"="Return the values of the power dynamics traces. Each value is sampled with 48 Ts, corresponding to 1.5625 s. The results of the maximum trace is retrieved.\n\nReturn values:  \n<Reliability>\n decimal\n\n<Power>\n float\n2048 power values, from -1100 s to +2098.4375 s relative to the start of the measure subframe. The values have a spacing of 1.5625 s. The 705th value is at the start of the 'Measure Subframe' (0 s).\nThe diagram in the GUI shows only a subsection of this trace.\nDefault unit:  dBm\n\nAvailable Repeated Capabilities:\ninstance: i0, i1, i2, i3, i4, i5, i6, i7, i8, i9, i10, i11, i12, i13, i14, i15, i16, i17, i18, i19, i20, i21, i22, i23, i24, i25, i26, i27, i28, i29, i30, i31, i32\r\n\nRemote-control command(s):\nFETCh:NRSub:MEAS<i>:MEValuation:TRACe:PDYNamics:MAXimum?"}, {"Level"=4, "Class Only"=FALSE, "Identifier"="RSCMWXPNRFR1M_ATTR_READ_MULTI_EVAL_MEAS_POWER_DYNAMICS_CURRENT_RESULTS", "Descriptive Name"="Read Multi Eval Meas Power Dynamics Current Results", "Data Type"=enum."RawString", "Command"="READ:NRS:MEAS{instance}:MEV:PDYN:CURR?", "Access"=enum."Read Only", "Range Table"="", "Read Callback"="", "Write Callback"="", "Range Callback"="", "Check Callback"="", "Rngtable Callback"="", "Coerce Callback"="", "Supported Models"="", "Instrument Options"="", "Check Status Callback"="", "Flags"=0, "Help"="Return the current single value results of the power dynamics measurement.\n\nReturn values:  \n<Reliability>\n decimal\n\n<OutOfTolerance>\n decimal\nOut of tolerance result, i.e. percentage of measurement intervals of the statistic count for power dynamics measurements 
